vi "TimeThreshold.vi"(2 "Threshold":dbl, 3 "Current Value":dbl) -> (0 "Time Below Threshold (ms)":u32, 1 "Time Above Threshold (ms)":u32)   [LabVIEW 2019]
doc: "Reports the time (in milliseconds) that the Current Value has been above or below the Threshold. If the Current Value is exaclty equal to the Threshold, both times output zero."
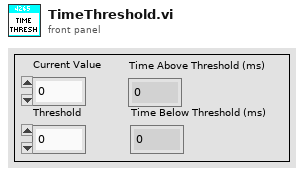
[diagram p1: front panel]
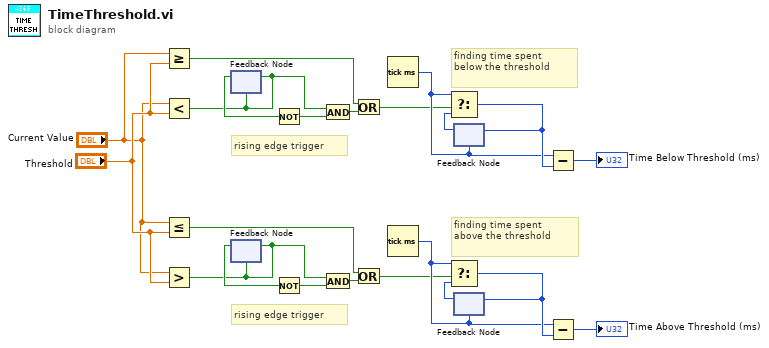
[diagram p0: block diagram]
diagram:
  # "rising edge trigger"
  # "finding time spent  \nabove the threshold"
  # "rising edge trigger"
  # "finding time spent  \nbelow the threshold"
  n1 = Greater Or Equal?(x="Current Value", y="Threshold") -> (x >= y?=w17:bool)
  n2 = Less?(x="Current Value", y="Threshold") -> (x < y?=w13:bool)
  n3 = Less Or Equal?(x="Current Value", y="Threshold") -> (x <= y?=w7:bool)
  n4 = Greater?(x="Current Value", y="Threshold") -> (0:w3:bool)
  n5 = feedback #1(w13) -> (w14:bool)
  n6 = feedback-in #1(w13) -> ()
  n7 = feedback #2(w3) -> (w4:bool)
  n8 = feedback-in #2(w3) -> ()
  n9 = Not(x=w14) -> (.not. x?=w16:bool)
  n10 = Not(x=w4) -> (.not. x?=w6:bool)
  n11 = And(x=w13, y=w16) -> (x .and. y?=w15:bool)
  n12 = And(x=w3, y=w6) -> (x .and. y?=w5:bool)
  n13 = Or(x=w17, y=w15) -> (x .or. y?=w18:bool)
  n14 = Or(x=w7, y=w5) -> (x .or. y?=w8:bool)
  n15 = Tick Count (ms)() -> (millisecond timer value=w20:u32)
  n16 = Tick Count (ms)() -> (millisecond timer value=w10:u32)
  n17 = feedback #3(w20) -> (w22:u32)
  n18 = Select(t=w20, s=w18, f=w22) -> (s? t:f=w21:u32)
  n19 = feedback-in #3(w21) -> ()
  n20 = feedback #4(w10) -> (w12:u32)
  n21 = Select(t=w10, s=w8, f=w12) -> (s? t:f=w11:u32)
  n22 = feedback-in #4(w11) -> ()
  n23 = Subtract(x=w20, y=w21) -> (x-y=→"Time Below Threshold (ms)":u32)
  n24 = Subtract(x=w10, y=w11) -> (x-y=→"Time Above Threshold (ms)":u32)
